vi "Daten Erfassung QSM.vi"(8 "error in":errorcluster, 9 "Daten-Queue (Eingang)":refnum<queue>, 10 "Nachrichten-Queues (Eingang)":T1) -> (0 "error out":errorcluster)   [LabVIEW 2014]
uses:
  All Message Queues.ctl
  Documents/LabVIEW Data/Unbenanntes Projekt 8/support/Message Queue/Message Cluster.ctl
  Documents/LabVIEW Data/Unbenanntes Projekt 8/support/Message Queue/Enqueue Message (Single).vi
  Documents/LabVIEW Data/Unbenanntes Projekt 8/support/Message Queue/Message Queue.lvlib
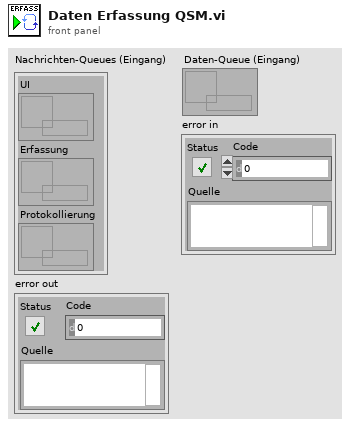
[diagram p1: front panel]
types:
  T1 = typedef "Message Queue.lvlib/All Message Queues.ctl" = cluster{"UI":refnum<queue>, "Erfassung":refnum<queue>, "Traverse":refnum<queue>}
  T2 = cluster{"Status":bool, "Code":i32, "Quelle":string}
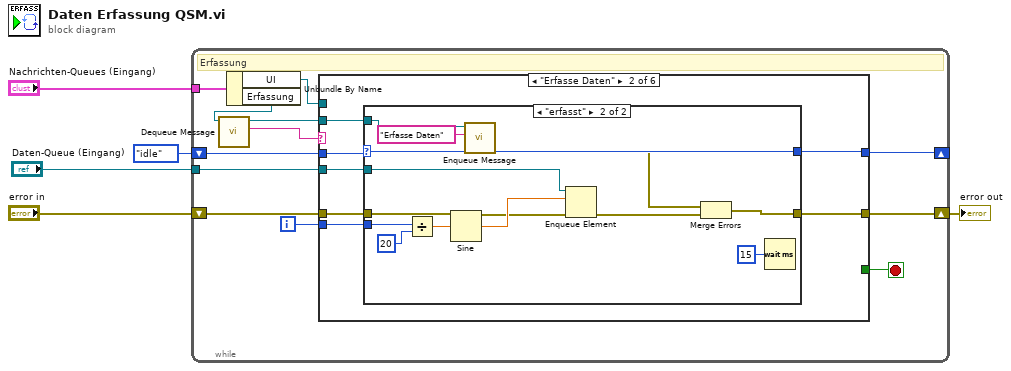
[diagram p0: block diagram]
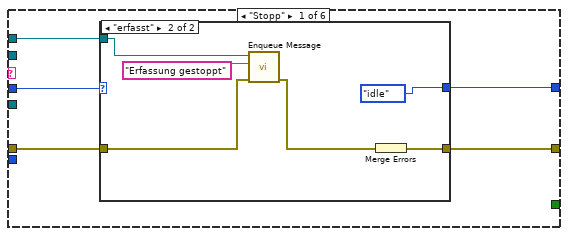
[diagram p2: hidden frame]
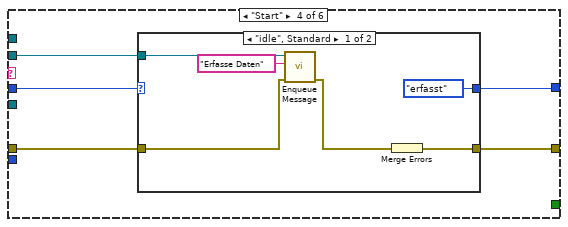
[diagram p6: hidden frame]
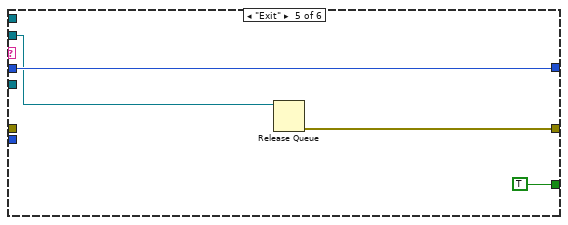
[diagram p8: hidden frame]
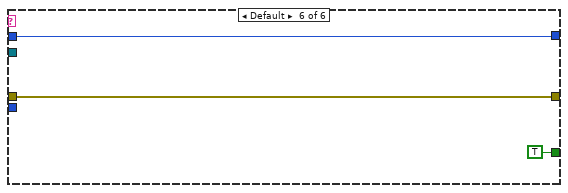
[diagram p9: hidden frame]
diagram:
  n1 = while {
    tunnel: "Daten-Queue (Eingang)" -> [w17]
    shift-right: [w14] -> _
    shift-left: enum16{"idle", "erfasst"}."idle" -> [w15]
    shift-right: [w11] -> w1
    shift-left: "error in" -> [w9]
    tunnel: "Nachrichten-Queues (Eingang)" -> [w6]
    i -> [w10]
    stop <- w12 stop-if-true
    # "Erfassung"
    n2 = Unbundle By Name(w6) -> ("UI"=w8:refnum<queue>, "Erfassung"=w7:refnum<queue>)
    n3 = call "Dequeue Message.vi"("Nachrichten-Queue"=w7) -> ("Nachricht"=w16:string, "Nachrichten-Queue (Kopie)"=w13:refnum<queue>)  [unwired: 7 in, 2 out]
    n4 = case shown="\"Erfasse Daten\"" w16 {
      tunnel: w17 -> [_ w35 _ _ _ _]
      tunnel: w15 -> [w22 w37 w54 w59 w70 w74]
      tunnel: [w21 w34 w54 w58 w70 w74] -> w14
      tunnel: w13 -> [_ w36 _ w57 w68 _]
      tunnel: w8 -> [w20 _ _ _ _ _]
      tunnel: [_ _ _ _ TRUE TRUE] -> w12
      tunnel: [w18 w31 w53 w56 w69 w72] -> w11
      tunnel: w10 -> [_ w33 _ _ _ _]
      tunnel: w9 -> [w19 w32 w53 w55 _ w72]
      frame "Stopp" {
        n5 = case shown="\"erfasst\"" w22 {
          selector: w22 -> [w24 _]
          tunnel: [w24 enum16{"idle", "erfasst"}."idle"] -> w21
          tunnel: w20 -> [_ w28]
          tunnel: w19 -> [w23 w27]
          tunnel: [w23 w25] -> w18
          frame "idle", Default {
          }
          frame "erfasst" {
            n6 = call-poly "Enqueue Message.vi"("error in (no error)"=w27, "Nachricht"="Erfassung gestoppt", "Nachrichten-Queue"=w28) -> ("error out"=w26:T2)  [unwired: 7 in, 1 out]
            n7 = Merge Errors(w26) -> (w25:errorcluster)
          }
        }
      }
      frame "Erfasse Daten" {
        n8 = case shown="\"erfasst\"" w37 {
          selector: w37 -> [w39 w49]
          tunnel: [w39 w49] -> w34
          tunnel: w36 -> [_ w48]
          tunnel: w35 -> [_ w46]
          tunnel: w33 -> [_ w44]
          tunnel: w32 -> [w38 w43]
          tunnel: [w38 w40] -> w31
          frame "idle", Default {
          }
          frame "erfasst" {
            n9 = Divide(x=w44, y=20) -> (x/y=w51:dbl)
            n10 = Sine(x=w51) -> (sin(x)=w45:dbl)
            n11 = call-poly "Enqueue Message.vi"("Nachricht"="Erfasse Daten", "Nachrichten-Queue"=w48) -> ("error out"=w42:T2)  [unwired: 8 in, 1 out]
            n12 = Enqueue Element(queue=w46, element=w45, error in (no error)=w43) -> (error out=w41:errorcluster)  [unwired: 1 in, 2 out]
            n13 = Merge Errors(w42, w41) -> (w40:errorcluster)
            n14 = Wait (ms)(milliseconds to wait=u32 15 ("Zu wartende ms")) -> ()  [unwired: 1 out]
          }
        }
      }
      frame "Initialize" {
      }
      frame "Start" {
        n15 = case shown="\"idle\", Standard" w59 {
          selector: w59 -> [_ w67]
          tunnel: [enum16{"idle", "erfasst"}."erfasst" w67] -> w58
          tunnel: w57 -> [w65 _]
          tunnel: [w61 w66] -> w56
          tunnel: w55 -> [w60 w66]
          frame "idle", Default {
            n16 = call-poly "Enqueue Message.vi"("error in (no error)"=w60, "Nachricht"="Erfasse Daten", "Nachrichten-Queue"=w65) -> ("error out"=w62:T2)  [unwired: 7 in, 1 out]
            n17 = Merge Errors(w62) -> (w61:errorcluster)
          }
          frame "erfasst" {
          }
        }
      }
      frame "Exit" {
        n18 = Release Queue(queue=w68) -> (error out=w69:errorcluster)  [unwired: 2 in, 2 out]
      }
      frame Default {
      }
    }
  }
  "error out" <- w1
